vi "GetCurrent.vi"(4 "error in":errorcluster, 5 "connection ID":refnum<k5>) -> (0 "Current":string, 1 "error out":errorcluster, 2 "connection ID out":refnum<k5>, 3 "Answer":bool)   [LabVIEW 2013]
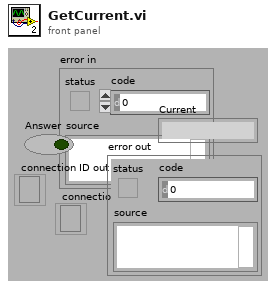
[diagram p1: front panel]
types:
  T1 = enum16{"Standard", "Buffered", "CRLF", "Immediate"}
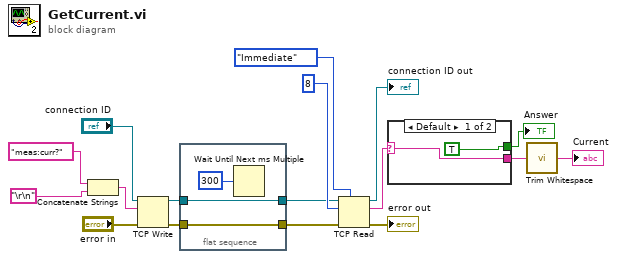
[diagram p0: block diagram]
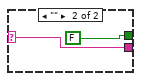
[diagram p2: hidden frame]
diagram:
  n1 = Concatenate Strings("meas:curr?" ("data in"), "\r\n") -> (w1:string)
  n2 = TCP Write(connection ID="connection ID", data in=w1, error in (no error)="error in") -> (connection ID out=w7:refnum<k5>, error out=w5:errorcluster)  [unwired: 2 out]
  n3 = flat-sequence {
    tunnel: w7 -> [w20]
    tunnel: [w20] -> w6
    tunnel: w5 -> [w19]
    tunnel: [w19] -> w4
    frame #0 {
      n4 = Wait Until Next ms Multiple(millisecond multiple=u32 300) -> ()  [unwired: 1 out]
    }
  }
  n5 = TCP Read(connection ID=w6, bytes to read=8, error in (no error)=w4, 7:T1."Immediate" ("mode (standard)")) -> (connection ID out=→"connection ID out":refnum<k5>, data out=w14:string, error out=→"error out":errorcluster)  [unwired: 1 out]
  n6 = case shown="Default" w14 {
    selector: w14 -> [w22 w24]
    tunnel: [w22 w24] -> w9
    tunnel: [TRUE FALSE] -> w13
    frame Default {
    }
    frame "" {
    }
  }
  "Answer" <- w13
  n7 = call <vilib>:"Trim Whitespace.vi"("string"=w9) -> ("trimmed string"=→"Current":string)  [unwired: 1 in]
